vi "move_relative.vi"(0 "VISA Refnum in":refnum<visa-resource-name>, 5 "Position":i32, 11 "error in (no error)":errorcluster) -> (4 "VISA Refnum out":refnum<visa-resource-name>, 15 "error out":errorcluster)   [LabVIEW 2020]
panel:
  out "read buffer":string
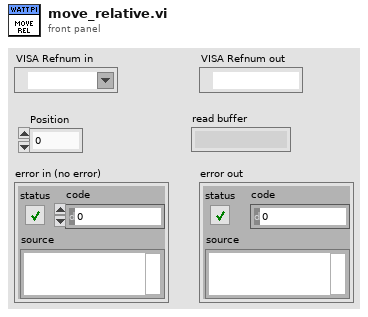
[diagram p1: front panel]
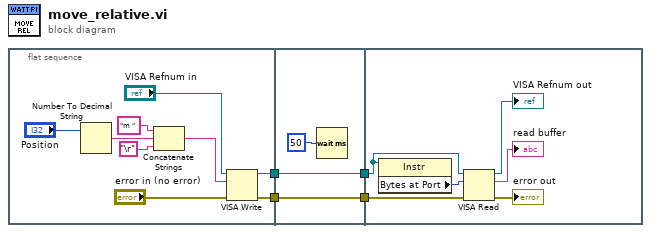
[diagram p0: block diagram]
diagram:
  n1 = flat-sequence {
    tunnel: [w13] -> w4
    tunnel: [w10] -> w3
    tunnel: w4 -> [w16]
    tunnel: w3 -> [w14]
    tunnel: [w16] -> w2
    tunnel: [w14] -> w1
    tunnel: w2 -> [w21]
    tunnel: w1 -> [w17]
    frame #0 {
      n2 = Number To Decimal String(number="Position") -> (decimal integer string=w6:string)  [unwired: 1 in]
      n3 = Concatenate Strings("m " ("write buffer"), w6, "\r") -> (w9:string)
      n4 = VISA Write(VISA resource name="VISA Refnum in", write buffer=w9, error in (no error)="error in (no error)") -> (VISA resource name out=w10:refnum<visa-resource-name>, error out=w13:errorcluster)  [unwired: 1 out]
    }
    frame #1 {
      n5 = Wait (ms)(milliseconds to wait=u32 50) -> ()  [unwired: 1 out]
    }
    frame #2 {
      n6 = property class="Instr"(reference=w17) -> ("Bytes at Port"=w18:u32)  [unwired: 1 in, 2 out]
      n7 = VISA Read(VISA resource name=w17, byte count=w18, error in (no error)=w21) -> (VISA resource name out=→"VISA Refnum out":refnum<visa-resource-name>, read buffer=→"read buffer":string, error out=→"error out":errorcluster)  [unwired: 1 out]
    }
  }
